vi "Read configuration.vi"(8 "error in":errorcluster, 11 "AppStateMachine editor node in":refnum<class "AppStateMachine editor node.lvclass">) -> (0 "error out":errorcluster, 2 "configuration":refnum<class "NISE_CEF_serializable configuration.lvclass">, 3 "AppStateMachine editor node out":refnum<class "AppStateMachine editor node.lvclass">)   [LabVIEW 2017, in "AppStateMachine editor node.lvclass"]
uses:
  AppStateMachine editor node.lvclass
  <vilib>/NI/Configuration Framework/serializable configuration/NISE_CEF_serializable configuration.lvclass
  AppStateMachine editor node.lvclass/AppStateMachine editor node.ctl
  module/configuration/AppStateMachine configuration.lvclass
  C:/Program Files (x86)/National Instruments/LabVIEW 2017/vi.lib/NI/Configuration Framework/serializable configuration/NISE_CEF_serializable configuration.lvclass
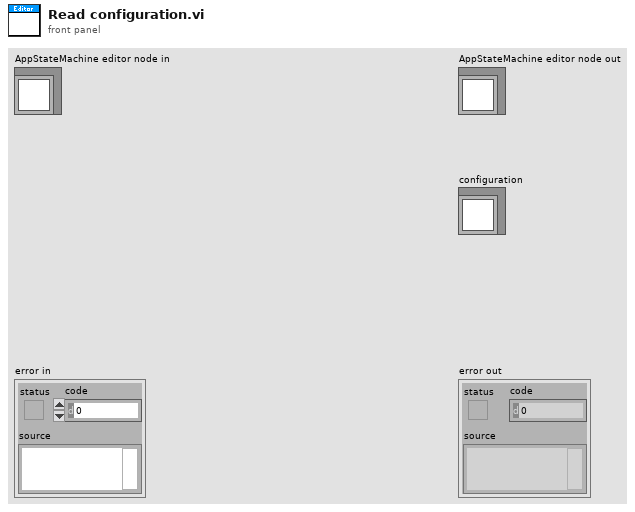
[diagram p1: front panel]
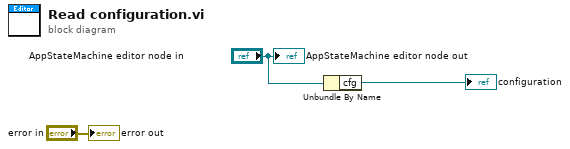
[diagram p0: block diagram]
diagram:
  n1 = Unbundle By Name("AppStateMachine editor node in") -> ("cfg"=→"configuration":refnum<class "AppStateMachine configuration.lvclass">)
  "error out" <- "error in"
  "AppStateMachine editor node out" <- "AppStateMachine editor node in"
